vi "Add FPGA Sections.vi"(8 "error in (no error)":errorcluster, 11 "Node Ptr":T1 format="%.0x") -> (0 "error out":errorcluster, 3 "Parent Ref out":T1 format="%.0x")   [LabVIEW 2018, in "FPGA Addon System Explorer.lvlib"]
uses:
  FPGA Addon System Explorer.lvlib
  <vilib>/NI Veristand/Custom Device API/Custom Device Item Ref.ctl
  Addon Shared/SubVIs/Constants.vi
  <vilib>/NI Veristand/Custom Device API/Custom Device API.lvlib
  Addon Shared/FPGA Addon Shared.lvlib
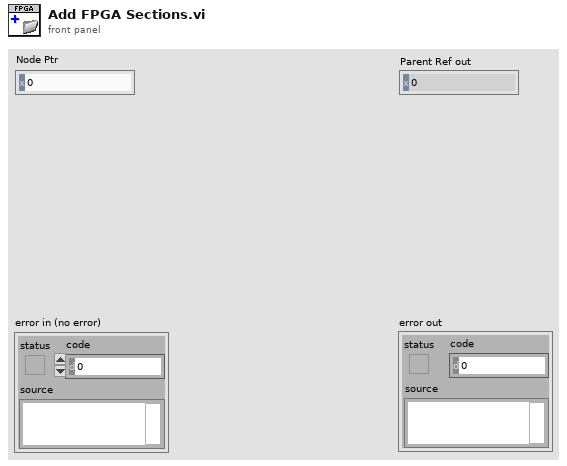
[diagram p1: front panel]
types:
  T1 = typedef "Custom Device API.lvlib/Custom Device Item Ref.ctl" = u64
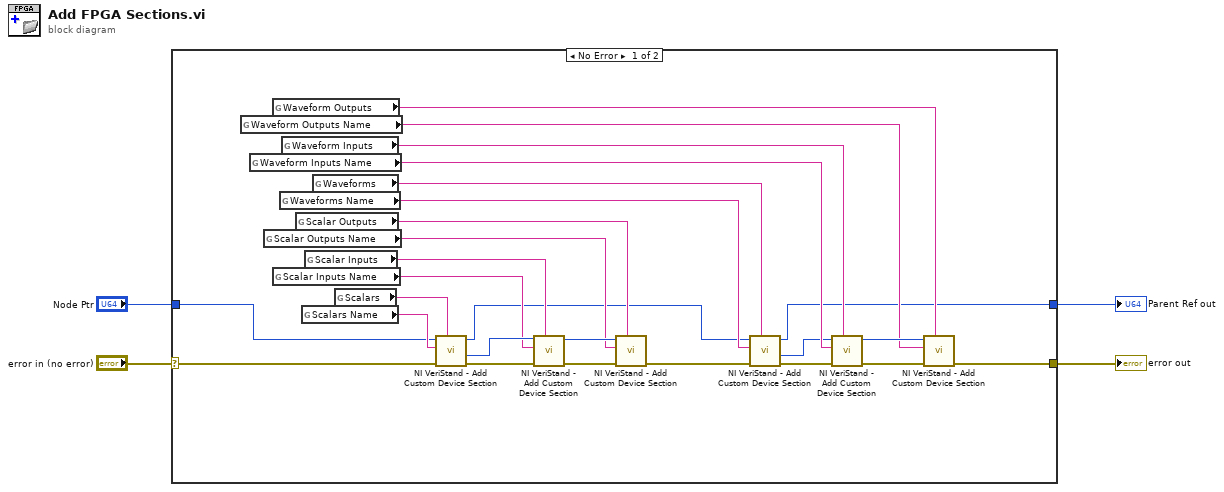
[diagram p0: block diagram]
diagram:
  n1 = case shown="No Error" "error in (no error)" {
    selector: "error in (no error)" -> [w5 w32]
    tunnel: [w8 w32] -> w4
    tunnel: [w7 w31] -> w3
    tunnel: "Node Ptr" -> [w6 w31]
    frame No Error {
      n2 = global read "Constants.vi" "Waveform Outputs Name"() -> (w10:string)
      n3 = global read "Constants.vi" "Waveform Inputs Name"() -> (w17:string)
      n4 = global read "Constants.vi" "Scalar Outputs Name"() -> (w22:string)
      n5 = global read "Constants.vi" "Waveform Outputs"() -> (w9:string)
      n6 = global read "Constants.vi" "Scalar Inputs Name"() -> (w26:string)
      n7 = global read "Constants.vi" "Waveforms Name"() -> (w20:string)
      n8 = global read "Constants.vi" "Waveform Inputs"() -> (w16:string)
      n9 = global read "Constants.vi" "Scalar Outputs"() -> (w21:string)
      n10 = global read "Constants.vi" "Scalars Name"() -> (w29:string)
      n11 = global read "Constants.vi" "Scalar Inputs"() -> (w25:string)
      n12 = global read "Constants.vi" "Waveforms"() -> (w19:string)
      n13 = global read "Constants.vi" "Scalars"() -> (w30:string)
      n14 = call <vilib>:"NI VeriStand - Add Custom Device Section.vi"("GUID (Default Section)"=w30, "error in (no error)"=w5, "Section Name"=w29, "Parent Ref in"=w6) -> ("error out"=w28:errorcluster, "Section Ptr"=w27:T1, "Parent Ref out"=w15:T1)  [unwired: 4 in, 1 out]
      n15 = call <vilib>:"NI VeriStand - Add Custom Device Section.vi"("GUID (Default Section)"=w25, "error in (no error)"=w28, "Section Name"=w26, "Parent Ref in"=w27) -> ("error out"=w23:errorcluster, "Parent Ref out"=w24:T1)  [unwired: 4 in, 2 out]
      n16 = call <vilib>:"NI VeriStand - Add Custom Device Section.vi"("GUID (Default Section)"=w21, "error in (no error)"=w23, "Section Name"=w22, "Parent Ref in"=w24) -> ("error out"=w14:errorcluster)  [unwired: 4 in, 3 out]
      n17 = call <vilib>:"NI VeriStand - Add Custom Device Section.vi"("GUID (Default Section)"=w19, "error in (no error)"=w14, "Section Name"=w20, "Parent Ref in"=w15) -> ("error out"=w18:errorcluster, "Section Ptr"=w11:T1, "Parent Ref out"=w7:T1)  [unwired: 4 in, 1 out]
      n18 = call <vilib>:"NI VeriStand - Add Custom Device Section.vi"("GUID (Default Section)"=w16, "error in (no error)"=w18, "Section Name"=w17, "Parent Ref in"=w11) -> ("error out"=w12:errorcluster, "Parent Ref out"=w13:T1)  [unwired: 4 in, 2 out]
      n19 = call <vilib>:"NI VeriStand - Add Custom Device Section.vi"("GUID (Default Section)"=w9, "error in (no error)"=w12, "Section Name"=w10, "Parent Ref in"=w13) -> ("error out"=w8:errorcluster)  [unwired: 4 in, 3 out]
    }
    frame Error {
    }
  }
  "error out" <- w4
  "Parent Ref out" <- w3
